vi "Button Press.vi"(1 "Current Button":bool) -> (0 "Pressed?":bool)   [LabVIEW 2017]
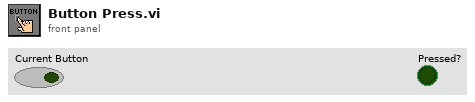
[diagram p1: front panel]
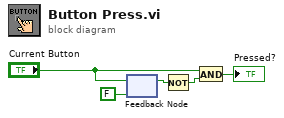
[diagram p0: block diagram]
diagram:
  n1 = feedback-in #1("Current Button") -> ()
  n2 = feedback #1(FALSE) -> (w4:bool)
  n3 = Not(x=w4) -> (.not. x?=w3:bool)
  n4 = And(x="Current Button", y=w3) -> (x .and. y?=→"Pressed?":bool)
